vi "Results_filename_checker.vi"(5 "Warn if Already Exists":bool, 6 "Comment":string, 7 "Show Error handler":bool=TRUE, 8 "Results file":path) -> (0 "exists?":bool, 1 "Error String":string, 2 "cancelled":bool, 3 "Results file output":path)   [LabVIEW 2020]
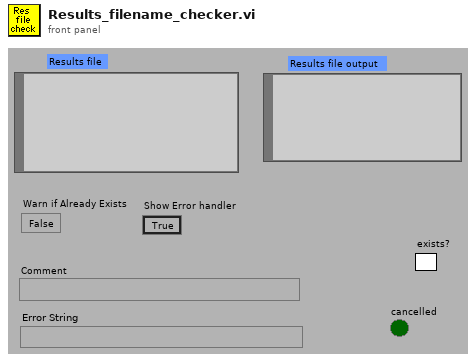
[diagram p1: front panel]
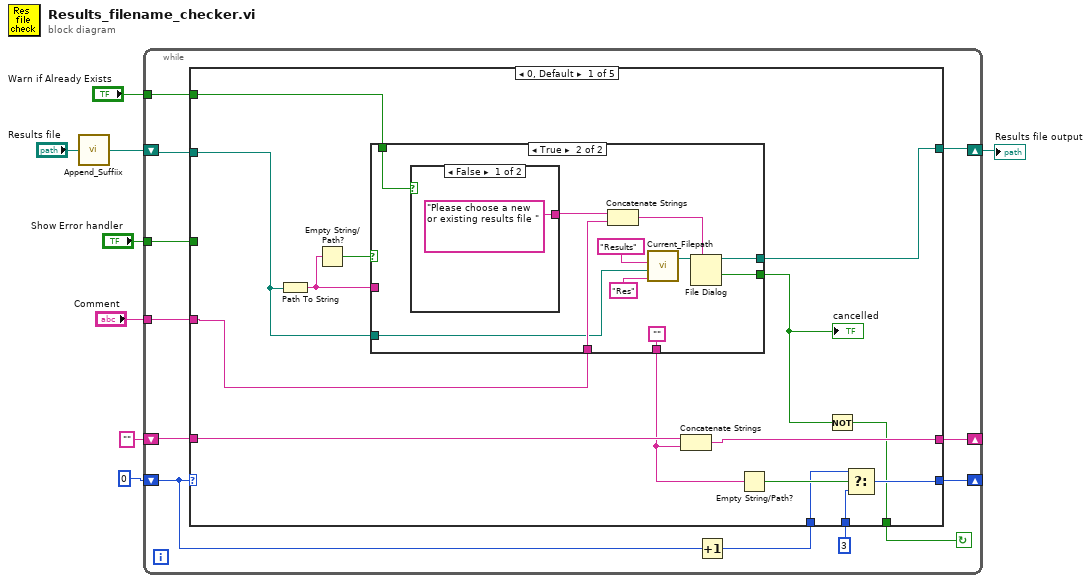
[diagram p0: block diagram]
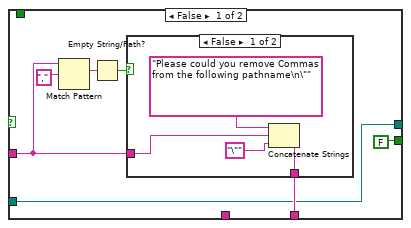
[diagram p2: hidden frame]
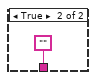
[diagram p3: hidden frame]
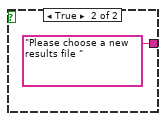
[diagram p4: hidden frame]
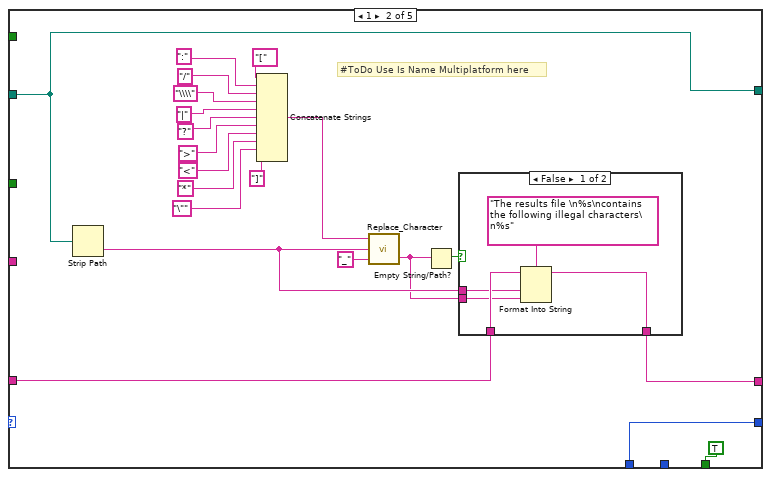
[diagram p5: hidden frame]
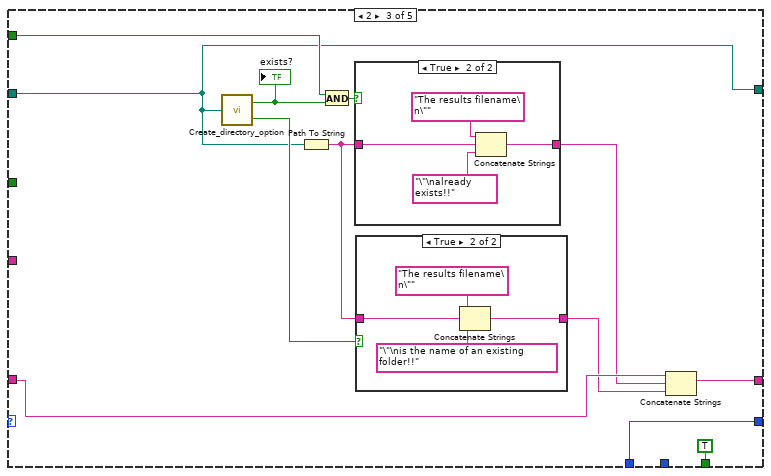
[diagram p7: hidden frame]
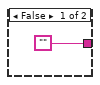
[diagram p8: hidden frame]
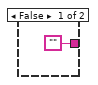
[diagram p9: hidden frame]
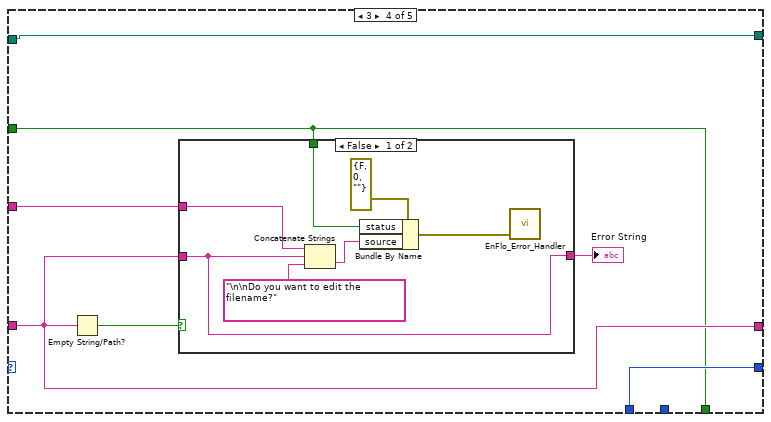
[diagram p10: hidden frame]
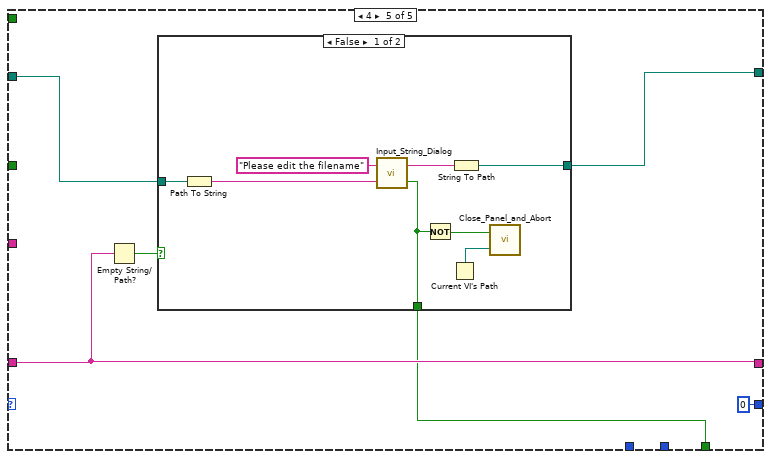
[diagram p12: hidden frame]
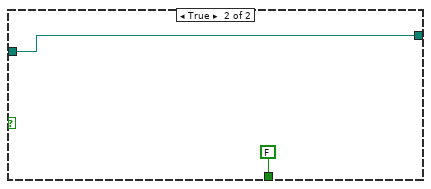
[diagram p13: hidden frame]
diagram:
  n1 = call "Append_Suffiix.vi"("Results file"="Results file") -> ("appended path"=w2:path)
  n2 = while {
    shift-left: 0 -> [w16]
    shift-right: [w12] -> _
    shift-left: "" -> [w15]
    shift-right: [w14] -> _
    tunnel: "Show Error handler" -> [w17]
    shift-left: w2 -> [w20]
    shift-right: [w19] -> w8
    tunnel: "Warn if Already Exists" -> [w11]
    tunnel: "Comment" -> [w10]
    stop <- w18 continue-if-true
    n3 = Increment(x=w16) -> (x+1=w13:i32)
    n4 = case shown="0, Default" w16 {
      tunnel: w20 -> [w28 w68 w89 w111 w129]
      tunnel: [w29 w68 w89 w111 w130] -> w19
      tunnel: [w25 TRUE ("Ok Out") TRUE ("Ok Out") w112 w127] -> w18
      tunnel: w17 -> [_ _ _ w112 _]
      tunnel: w15 -> [w35 w66 w96 w114 w128]
      tunnel: [w34 w65 w95 w114 w128] -> w14
      tunnel: w13 -> [w31 w64 w93 w113 _]
      tunnel: [w30 w64 w93 w113 0 ("f")] -> w12
      tunnel: w11 -> [w27 _ w90 _ _]
      tunnel: w10 -> [w24 _ _ w110 _]
      tunnel: 3 ("f") -> [w23 _ _ _ _]
      frame 0, Default {
        n5 = Path To String(path=w28) -> (string=w22:string)
        n6 = Empty String/Path?(string/path=w22) -> (empty?=w21:bool)
        n7 = case shown="True" w21 {
          tunnel: [w42 ""] -> w33
          tunnel: w22 -> [w38 _]
          tunnel: [w37 w53] -> w29
          tunnel: w28 -> [w37 w50]
          tunnel: w27 -> [_ w57]
          tunnel: [FALSE ("cancelled") w52] -> w26
          tunnel: w24 -> [_ w55]
          frame False {
            n8 = Match Pattern(string=w38, regular expression=",") -> (match substring=w40:string)  [unwired: 4 out]
            n9 = Empty String/Path?(string/path=w40) -> (empty?=w39:bool)
            n10 = case shown="False" w39 {
              tunnel: w38 -> [w45 _]
              tunnel: [w44 ""] -> w42
              frame False {
                n11 = Concatenate Strings("Please could you remove Commas from the following pathname\n\"", w45, "\"") -> (w44:string)
              }
              frame True {
              }
            }
          }
          frame True {
            n12 = case shown="False" w57 {
              tunnel: ["Please choose a new or existing results file " ("prompt") "Please choose a new results file " ("prompt")] -> w56
              frame False {
              }
              frame True {
              }
            }
            n13 = Concatenate Strings(w56, w55) -> (w54:string)
            n14 = call "Current_Filepath.vi"("Short_Name"="Res" ("Data Type"), "Filename in"=w50, "Data Type"="Results") -> ("Directory"=w49:path)  [unwired: 1 in, 1 out]
            n15 = File Dialog(7:w54, 11:w49) -> (1:w52:bool, 3:w53:path)  [unwired: 5 in, 2 out]
          }
        }
        "cancelled" <- w26
        n16 = Concatenate Strings(w35, w33) -> (w34:string)
        n17 = Empty String/Path?(string/path=w33) -> (empty?=w32:bool)
        n18 = Not(x=w26) -> (.not. x?=w25:bool)
        n19 = Select(t=w31, s=w32, f=w23) -> (s? t:f=w30:i32)
      }
      frame 1 {
        # "#ToDo Use Is Name Multiplatform here"
        n20 = Strip Path(path=w68) -> (name=w62:string)  [unwired: 1 out]
        n21 = Concatenate Strings("[" ("Substring"), ":", "/", "\\\\", "|", "?", ">", "<", "*", "\"", "]" ("Substring")) -> (w70:string)
        n22 = call "Replace_Character.vi"("Replace with"="_", "Input String"=w62, "Search For"=w70) -> ("Matched Characters"=w61:string)  [unwired: 1 out]
        n23 = Empty String/Path?(string/path=w61) -> (empty?=w67:bool)
        n24 = case shown="False" w67 {
          tunnel: w66 -> [w85 w87]
          tunnel: [w84 w87] -> w65
          tunnel: w62 -> [w83 _]
          tunnel: w61 -> [w82 _]
          frame False {
            n25 = Format Into String(format string="The results file \n%s\ncontains the following illegal characters\n%s" ("Format String"), initial string=w85, w83, w82) -> (resulting string=w84:string)  [unwired: 1 in, 1 out]
          }
          frame True {
          }
        }
      }
      frame 2 {
        n26 = call "Create_directory_option.vi"("Filename"=w89) -> ("Path is to existing File"=w98:bool, "Path is to existing Directory"=w91:bool)
        "exists?" <- w98
        n27 = Path To String(path=w89) -> (string=w88:string)
        n28 = And(x=w90, y=w98) -> (x .and. y?=w97:bool)
        n29 = case shown="True" w97 {
          tunnel: ["" w107] -> w94
          tunnel: w88 -> [_ w106]
          frame False {
          }
          frame True {
            n30 = Concatenate Strings("The results filename\n\"", w106, "\"\nalready exists!!") -> (w107:string)
          }
        }
        n31 = case shown="True" w91 {
          tunnel: ["" w102] -> w92
          tunnel: w88 -> [_ w101]
          frame False {
          }
          frame True {
            n32 = Concatenate Strings("The results filename\n\"", w101, "\"\nis the name of an existing folder!!") -> (w102:string)
          }
        }
        n33 = Concatenate Strings(w96, w94, w92) -> (w95:string)
      }
      frame 3 {
        n34 = Empty String/Path?(string/path=w114) -> (empty?=w116:bool)
        n35 = case shown="False" w116 {
          tunnel: w114 -> [w118 w124]
          tunnel: [w118 w124] -> w115
          tunnel: w112 -> [w120 _]
          tunnel: w110 -> [w117 _]
          frame False {
            n36 = Concatenate Strings(w117, w118, "\n\nDo you want to edit the filename?") -> (w119:string)
            n37 = Bundle By Name(cluster=errorcluster {"status"=FALSE, "code"=0, "source"=""} ("error in (no error)"), "status"=w120, "source"=w119) -> (w122:errorcluster)
            n38 = call "EnFlo_Error_Handler.vi"("error in (no error)"=w122) -> ()  [unwired: 2 in, 3 out]
          }
          frame True {
          }
        }
        "Error String" <- w115
      }
      frame 4 {
        n39 = Empty String/Path?(string/path=w128) -> (empty?=w125:bool)
        n40 = case shown="False" w125 {
          tunnel: [w131 w139] -> w130
          tunnel: [w133 FALSE ("Ok Out")] -> w127
          tunnel: w129 -> [w136 w139]
          frame False {
            n41 = Path To String(path=w136) -> (string=w132:string)
            n42 = call "Input_String_Dialog.vi"("Value"=w132, "Message to user"="Please edit the filename") -> ("Ok Out"=w133:bool, "Output string"=w137:string)
            n43 = Not(x=w133) -> (.not. x?=w135:bool)
            n44 = Current VI's Path() -> (path=w134:path)
            n45 = String To Path(string=w137) -> (path=w131:path)
            n46 = call "Close_Panel_and_Abort.vi"("Vi path"=w134, "stop"=w135) -> ()  [unwired: 1 out]
          }
          frame True {
          }
        }
      }
    }
  }
  "Results file output" <- w8
